vi "Log Data.vi"(7 "Time Stamp":timestamp, 8 "error in":errorcluster, 9 "Data":variant, 10 "Ident":string, 11 "IData Logger Actor in":refnum<class "IData Logger Actor.lvclass">) -> (0 "error out":errorcluster, 3 "IData Logger Actor out":refnum<class "IData Logger Actor.lvclass">)   [LabVIEW 2023, in "IData Logger Actor.lvlib" / "IData Logger Actor.lvclass"]
uses:
  IData Logger Actor.lvclass
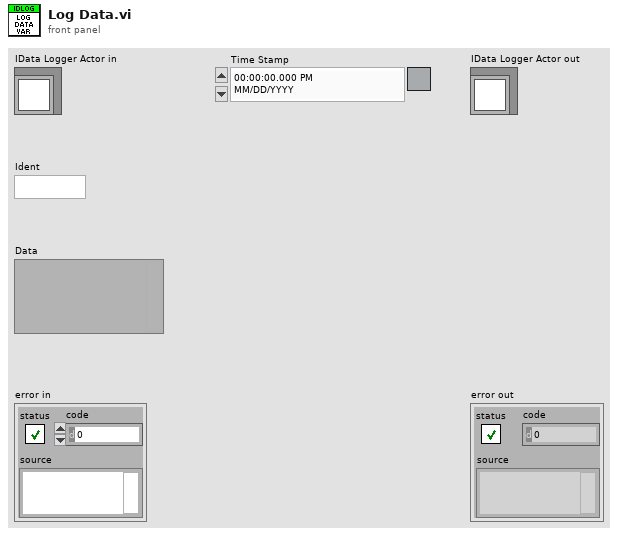
[diagram p1: front panel]
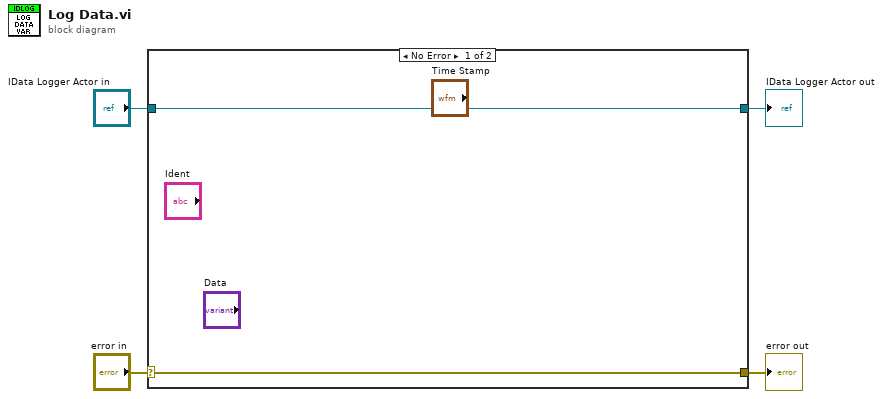
[diagram p0: block diagram]
diagram:
  n1 = case shown="No Error" "error in" {
    selector: "error in" -> [w5 w8]
    tunnel: [w5 w8] -> w3
    tunnel: [w6 w7] -> w1
    tunnel: "IData Logger Actor in" -> [w6 w7]
    frame No Error {
    }
    frame Error {
    }
  }
  "error out" <- w3
  "IData Logger Actor out" <- w1
